vi "instrumentProperties_channel_gainIndex_nr.vi"(8 "error in (no error)":errorcluster, 11 "OSAchannel in":refnum<class "OSAchannel.lvclass">) -> (0 "error out":errorcluster, 2 "levels_nr":u16, 3 "OSAchannel out":refnum<class "OSAchannel.lvclass">)   [LabVIEW 2010, in "OSAchannel.lvclass"]
uses:
  OSAchannel.lvclass
  OSAchannel.lvclass/OSAchannel.ctl
  FTSLib.dll
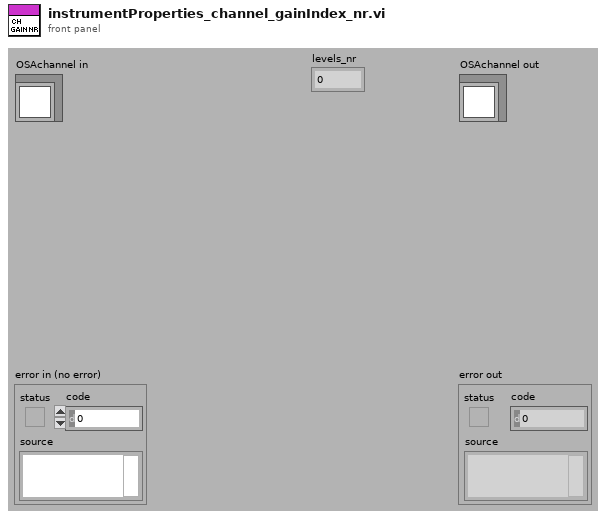
[diagram p1: front panel]
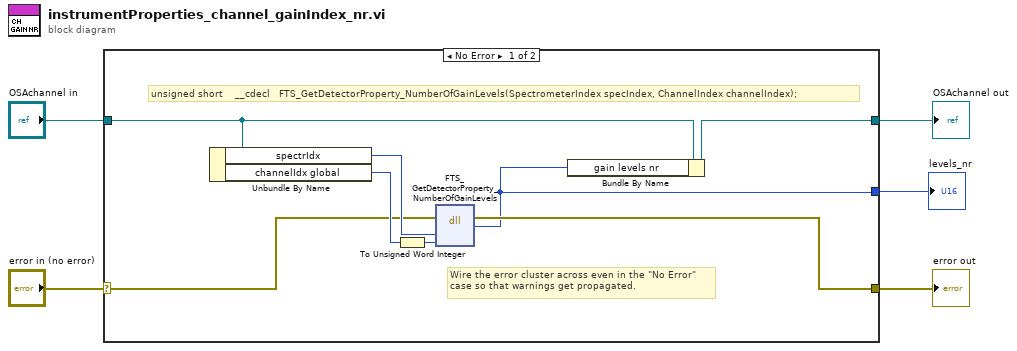
[diagram p0: block diagram]
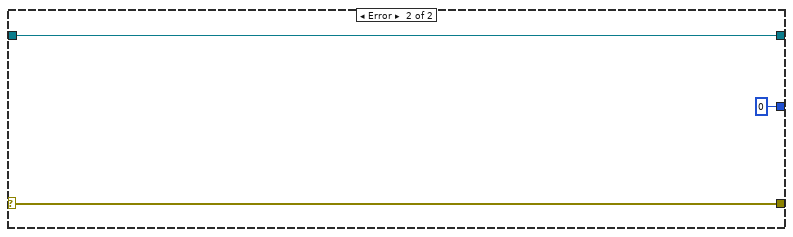
[diagram p2: hidden frame]
diagram:
  n1 = case shown="No Error" "error in (no error)" {
    selector: "error in (no error)" -> [w10 w16]
    tunnel: [w7 w16] -> w4
    tunnel: [w8 w15] -> w2
    tunnel: "OSAchannel in" -> [w9 w15]
    tunnel: [w6 u16 0 ("levels_nr")] -> w1
    frame No Error {
      # "unsigned short \t\t\t__cdecl   FTS_GetDetectorProperty_NumberOfGainLevels(SpectrometerIndex specIndex, ChannelIndex channelIndex);"
      # "Wire the error cluster across even in the \"No Error\"\ncase so that warnings get propagated."
      n2 = Unbundle By Name(w9) -> ("spectrIdx"=w13:u16, "channelIdx global"=w12:u16)
      n3 = To Unsigned Word Integer(number=w12) -> (unsigned 16bit integer=w11:u16)
      n4 = dll-call lib="FTSLib.dll" fn="FTS_GetDetectorProperty_NumberOfGainLevels"(error in=w10, "spectrIdx"=w13, "channeldx"=w11) -> (error out=w7:errorcluster, "levels_nr"=w6:u16)  [unwired: 4 in, 1 out]
      n5 = Bundle By Name(cluster=w9, "gain levels nr"=w6) -> (w8:refnum<class "OSAchannel.lvclass">)
    }
    frame Error {
    }
  }
  "error out" <- w4
  "OSAchannel out" <- w2
  "levels_nr" <- w1
